vi "Attenuator Close Test.vi"(6 "Driver Refs":T1, 8 "error in (no error)":errorcluster) -> (0 "error out":errorcluster {"code" format="%.0x"})   [LabVIEW 2011]
uses:
  TypeDefs/Attenuator Driver Refs.ctl
  drivers/ATT/ATT Driver Ref.ctl
  drivers/VNA/VNA Driver Ref.ctl
  drivers/SNA/SNA Driver Ref.ctl
  drivers/ATT/ATT Command.ctl
  drivers/VNA/VNA Command.ctl
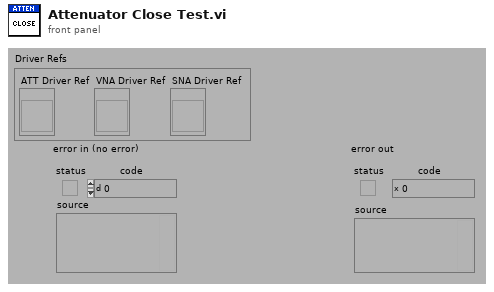
[diagram p1: front panel]
types:
  T1 = typedef "Attenuator Driver Refs.ctl" = cluster{"ATT Driver Ref":T2, "VNA Driver Ref":T3, "SNA Driver Ref":T4}
  T2 = typedef "ATT Driver Ref.ctl" = refnum<vi>
  T3 = typedef "VNA Driver Ref.ctl" = refnum<vi>
  T4 = typedef "SNA Driver Ref.ctl" = refnum<vi>
  T5 = typedef "VNA Command.ctl" = enum16{"LOAD", "INITIALIZE", "PRESET", "GET STIMULUS", "SET STIMULUS", "GET CALIBRATION", "CALIBRATE", "RESTORE", "MEASURE", "RELEASE", "UNLOAD", "CONFIRM", "SORT"}
  T6 = typedef "ATT Command.ctl" = enum16{"LOAD", "INITIALIZE", "PRESET", "SET STIMULUS", "GET STIMULUS", "GET CALIBRATION", "CALIBRATE", "GET INFO", "RELEASE", "UNLOAD"}
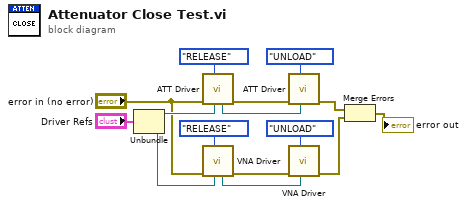
[diagram p0: block diagram]
diagram:
  n1 = Unbundle("Driver Refs") -> ("ATT Driver Ref"=w3:T2, "VNA Driver Ref"=w2:T3)  [unwired: 1 out]
  n2 = call "ATT Driver.vi"("Drv Refnum"=w3, "ATT Command"=ATT_Command."RELEASE" ("DMM Command"), "error in (no error)"="error in (no error)") -> ("error out"=w10:errorcluster, "dup Drv Refnum"=w8:T2)  [unwired: 5 in, 2 out]
  n3 = call "VNA Driver.vi"("Drv Refnum"=w2, "VNA Command"=VNA_Command."RELEASE", "error in (no error)"="error in (no error)") -> ("error out"=w11:errorcluster, "dup Drv Refnum"=w7:T3)  [unwired: 4 in, 3 out]
  n4 = call "ATT Driver.vi"("Drv Refnum"=w8, "ATT Command"=ATT_Command."UNLOAD" ("DMM Command"), "error in (no error)"=w10) -> ("error out"=w6:errorcluster)  [unwired: 5 in, 3 out]
  n5 = call "VNA Driver.vi"("Drv Refnum"=w7, "VNA Command"=VNA_Command."UNLOAD", "error in (no error)"=w11) -> ("error out"=w5:errorcluster)  [unwired: 4 in, 4 out]
  n6 = Merge Errors(w6, w5) -> (→"error out":errorcluster)
